vi "Servo Back and Forth(SubVI).vi"(0 "Upper Bound":i32, 1 "Original Value":i32, 2 "Increment in":bool, 3 "Lower Bound":i32) -> (7 "Increment out":bool, 8 "New Value":i32)   [LabVIEW 2017]
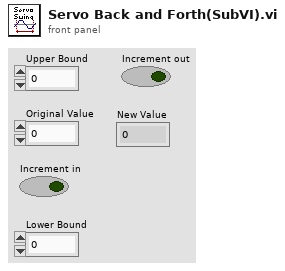
[diagram p1: front panel]
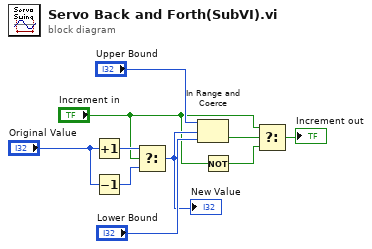
[diagram p0: block diagram]
diagram:
  n1 = Increment(x="Original Value") -> (x+1=w10:i32)
  n2 = Decrement(x="Original Value") -> (x-1=w9:i32)
  n3 = Select(t=w10, s="Increment in", f=w9) -> (s? t:f=w5:i32)
  "New Value" <- w5
  n4 = In Range and Coerce(upper limit="Upper Bound", x=w5, lower limit="Lower Bound") -> (In Range?=w4:bool)  [unwired: 1 out]
  n5 = Not(x="Increment in") -> (.not. x?=w2:bool)
  n6 = Select(t="Increment in", s=w4, f=w2) -> (s? t:f=→"Increment out":bool)
